vi "FastMap - Init.vi"() -> (3 "fast map out":refnum<data-value>)   [LabVIEW 2015, in "DS Square.lvlib"]
uses:
  DS Square.lvlib
  Square/Square.lvclass
  Square State Fast.ctl
  Fast Map.ctl
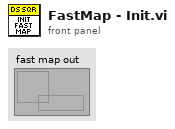
[diagram p1: front panel]
types:
  T1 = typedef "DS Square.lvlib/Fast Map.ctl" = cluster{"state":T2[][], "updated":i32[][]}
  T2 = typedef "DS Square.lvlib/Square State Fast.ctl" = enum8{"Unknown", "Empty", "Occupied - Active", "Occupied - Cool Down", "Attacked", "Enemy", "Enemy Wall"}
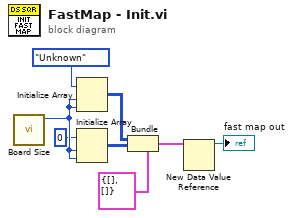
[diagram p0: block diagram]
diagram:
  n1 = call "Board Size.vi"() -> ("Board Size"=w8:i32)  [unwired: 11 in]
  n2 = Initialize Array(Square_State_Fast."Unknown" ("square state"), w8, w8) -> (w4:T2[][])
  n3 = Initialize Array(0, w8, w8) -> (w3:i32[][])
  n4 = Bundle(cluster=T1 {"state"=[], "updated"=[]} ("fast map data"), "state"=w4, "updated"=w3) -> (w2:T1)
  n5 = New Data Value Reference(data value=w2) -> (data value reference=→"fast map out":refnum<data-value>)  [unwired: 1 in, 1 out]
